vi "Replace Unflatten Types.vi"(4 "Fields":T1[](array[typedef]), 7 "Unflatten Refs":T4, 8 "error in (no error)":errorcluster, 9 "Bundlers":refnum<vi>[](array[refnum]), 10 "Decodes":refnum<vi>[](array[refnum]), 11 "LV-Protoc in":refnum<class "LV-Protoc.lvclass">) -> (0 "error out":errorcluster, 3 "LV-Protoc out":refnum<class "LV-Protoc.lvclass">)   [LabVIEW 2020, in "LV-Protoc.lvlib" / "LV-Protoc.lvclass"]
uses:
  LV-Protoc.lvclass
  Unflatten Refs.ctl
  LV-Proto/Field.ctl
  LV-Proto/Type.ctl
  LV-Proto/Proto Type.ctl
  LV-Proto/LV-Proto.lvlib
  LV-Protoc.lvlib
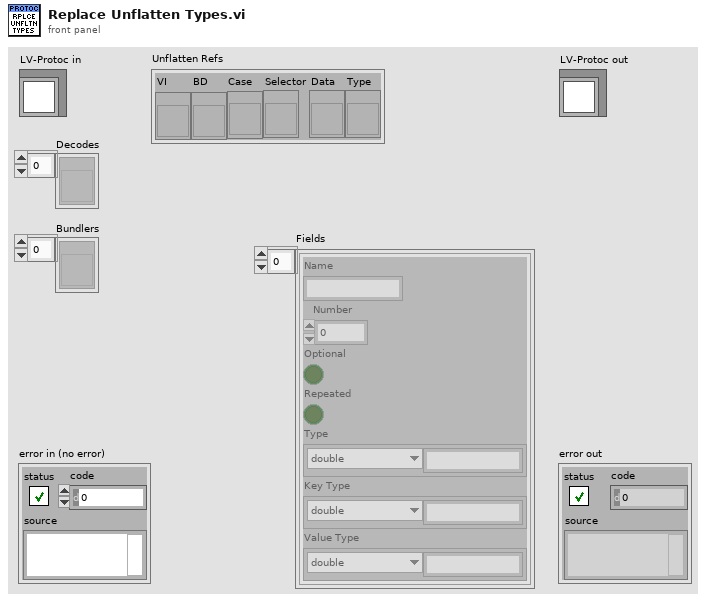
[diagram p1: front panel]
types:
  T1 = typedef "LV-Proto.lvlib/Field.ctl" = cluster{"Name":string, "Number":u32, "Optional":bool, "Repeated":bool, "Type":T2, "Key Type":T2, "Value Type":T2}
  T2 = typedef "LV-Proto.lvlib/Type.ctl" = cluster{"Type":T3, "Subtype":string}
  T3 = typedef "LV-Proto.lvlib/Proto Type.ctl" = enum16{"UNKNOWN", "double", "float", "int32", "int64", "uint32", "uint64", "sint32", "sint64", "fixed32", "fixed64", "sfixed32", "sfixed64", "bool", "string", "bytes", "enum", "map", "message"}
  T4 = typedef "LV-Protoc.lvlib/Unflatten Refs.ctl" = cluster{"VI":refnum<vi>, "BD":refnum<vi>, "Case":refnum<vi>, "Selector":refnum<vi>, "Data":refnum<vi>, "Type":refnum<vi>}
  T5 = typedef "LV-Protoc.lvlib/Enumeration Paths.ctl" = cluster{"Name":string, "Library":path, "Typedef":path, "Encode":path, "Encode packed":path, "Decode":path, "Decode packed":path, "Enum Value":path, "Enum from Value":path}
  T6 = typedef "LV-Protoc.lvlib/Message Paths.ctl" = cluster{"Name":string, "Library":path, "Data Typedef":path, "MessageName VI":path, "Flatten VI":path, "Unflatten VI":path, "Flatten repeated VI":path, "Decode VI":path}
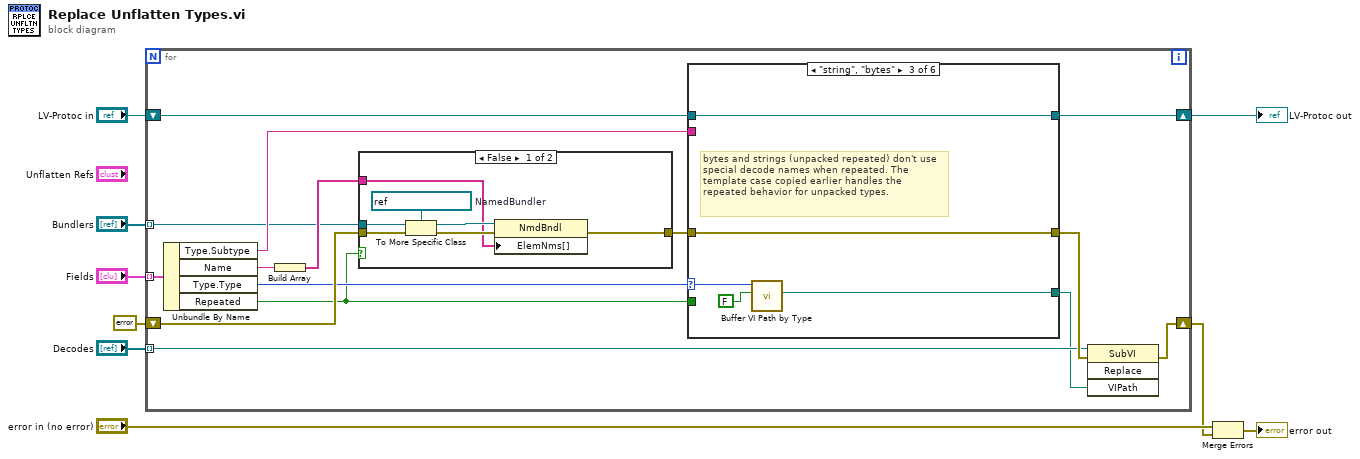
[diagram p0: block diagram]
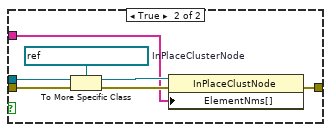
[diagram p2: hidden frame]
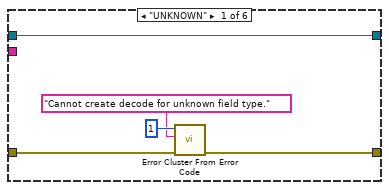
[diagram p3: hidden frame]
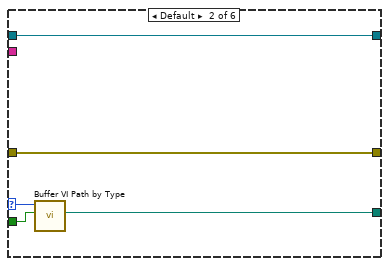
[diagram p4: hidden frame]
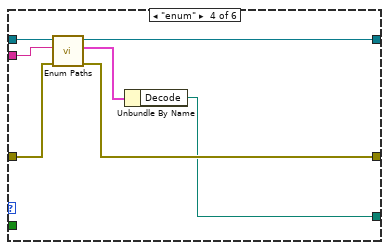
[diagram p5: hidden frame]
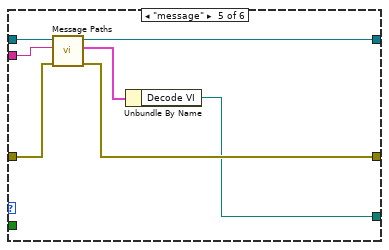
[diagram p6: hidden frame]
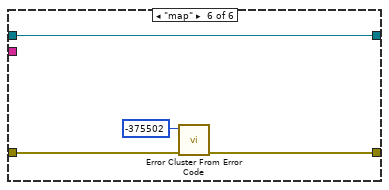
[diagram p7: hidden frame]
diagram:
  n1 = for {
    shift-right: [w19] -> w3
    shift-left: errorcluster {"status"=FALSE, "code"=0, "source"=""} ("error out") -> [w24]
    tunnel: "Decodes" -> [w20] mode=indexing
    tunnel: "Bundlers" -> [w11] mode=indexing
    tunnel: "Fields" -> [w21] mode=indexing
    shift-right: [w15] -> w5
    shift-left: "LV-Protoc in" -> [w16]
    n2 = Unbundle By Name(w21) -> ("Type.Subtype"=w14:string, "Name"=w10:string, "Type.Type"=w18:T3, "Repeated"=w13:bool)
    n3 = Build Array(w10) -> (w12:string[])
    n4 = case shown="False" w13 {
      tunnel: w12 -> [w26 w33]
      tunnel: w11 -> [w31 w38]
      tunnel: w24 -> [w29 w36]
      tunnel: [w25 w32] -> w23
      frame False {
        w30 = refnum<vi> refnum  # NamedBundler
        n5 = To More Specific Class(target class=w30, reference=w31, error in=w29) -> (specific class reference=w28:refnum<vi>, error out=w27:errorcluster)
        n6 = property class="NmdBndl"(reference=w28, error in=w27, "ElemNms[]"=w26) -> (error out=w25:errorcluster)  [unwired: 1 out]
      }
      frame True {
        w37 = refnum<vi> refnum  # InPlaceClusterNode
        n7 = To More Specific Class(target class=w37, reference=w38, error in=w36) -> (specific class reference=w35:refnum<vi>, error out=w34:errorcluster)
        n8 = property class="InPlaceClustNode"(reference=w35, error in=w34, "ElementNms[]"=w33) -> (error out=w32:errorcluster)  [unwired: 1 out]
      }
    }
    n9 = case shown="\"string\", \"bytes\"" w18 {
      selector: w18 -> [_ w47 w50 _ _ _]
      tunnel: w13 -> [_ w48 _ _ _ _]
      tunnel: [_ w46 w51 w54 w61 _] -> w17
      tunnel: w23 -> [w42 w44 w52 w56 w63 w70]
      tunnel: w16 -> [w43 w45 w53 w59 w66 w71]
      tunnel: [w43 w45 w53 w58 w65 w71] -> w15
      tunnel: [w41 w44 w52 w60 w67 w69] -> w22
      tunnel: w14 -> [_ _ _ w57 w64 _]
      frame "UNKNOWN" {
        n10 = call <vilib>:"Error Cluster From Error Code.vi"("error in (no error)"=w42, "error message (\"\")"="Cannot create decode for unknown field type.", "error code (0)"=1) -> ("error out"=w41:errorcluster)  [unwired: 6 in]
      }
      frame Default {
        n11 = call "Buffer VI Path by Type.vi"("Repeated"=w48, "Proto Type"=w47) -> ("Decode"=w46:path)  [unwired: 8 in, 1 out]
      }
      frame "string", "bytes" {
        # "bytes and strings (unpacked repeated) don't use special decode names when repeated. The template case copied earlier handles the repeated behavior for unpacked types."
        n12 = call "Buffer VI Path by Type.vi"("Repeated"=FALSE, "Proto Type"=w50) -> ("Decode"=w51:path)  [unwired: 8 in, 1 out]
      }
      frame "enum" {
        n13 = call "Enum Paths.vi"("error in (no error)"=w56, "Enum Type Name"=w57, "LV-Protoc in"=w59) -> ("error out"=w60:errorcluster, "Enum Paths"=w55:T5, "LV-Protoc out"=w58:refnum<class "LV-Protoc.lvclass">)  [unwired: 6 in]
        n14 = Unbundle By Name(w55) -> ("Decode"=w54:path)
      }
      frame "message" {
        n15 = call "Message Paths.vi"("error in (no error)"=w63, "Message Type Name"=w64, "LV-Protoc in"=w66) -> ("error out"=w67:errorcluster, "Message Paths"=w62:T6, "LV-Protoc out"=w65:refnum<class "LV-Protoc.lvclass">)  [unwired: 6 in]
        n16 = Unbundle By Name(w62) -> ("Decode VI"=w61:path)
      }
      frame "map" {
        n17 = call <vilib>:"Error Cluster From Error Code.vi"("error in (no error)"=w70, "error code (0)"=-375502) -> ("error out"=w69:errorcluster)  [unwired: 7 in]
      }
    }
    n18 = invoke class="SubVI" method="Replace"(reference=w20, error in=w22, "VIPath"=w17) -> (error out=w19:errorcluster)  [unwired: 1 in, 3 out]
  }
  "LV-Protoc out" <- w5
  n19 = Merge Errors("error in (no error)", w3) -> (→"error out":errorcluster)
